vi "S7-TCP_Close.vi"(8 "error in (no error)":errorcluster caption="错误输入（无错误）", 11 "S7-TCP 输入":refnum<class "S7-TCP.lvclass">) -> (0 "error out":errorcluster caption="错误输出")   [LabVIEW 2018, in "S7-TCP.lvclass"]
uses:
  S7-TCP.lvclass
  S7-TCP.lvclass/S7-TCP.ctl
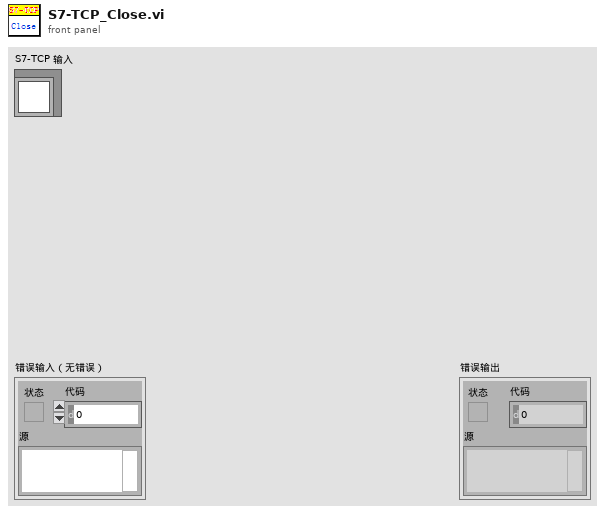
[diagram p1: front panel]
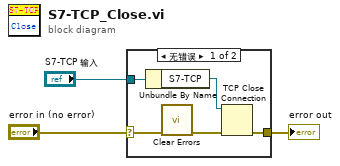
[diagram p0: block diagram]
diagram:
  n1 = case shown="无错误" "error in (no error)" {
    selector: "error in (no error)" -> [w6 w9]
    tunnel: [w5 w9] -> w2
    tunnel: "S7-TCP 输入" -> [w8 _]
    frame No Error {
      n2 = Unbundle By Name(w8) -> ("S7-TCP"=w7:refnum<k5>)
      n3 = call <vilib>:"Clear Errors.vi"("error in (no error)"=w6) -> ("error out"=w4:errorcluster)  [unwired: 5 in, 1 out]
      n4 = TCP Close Connection(connection ID=w7, error in (no error)=w4) -> (error out=w5:errorcluster)  [unwired: 1 in, 1 out]
    }
    frame Error {
    }
  }
  "error out" <- w2
